vi "Resolve IP.vi"(10 "error in (no error)":errorcluster, 11 "Address In":string) -> (2 "error out":errorcluster, 3 "U32 Address":u32 format="%08x", 5 "Address Type":T1)   [LabVIEW 2020, in "Vecto.lvlib"]
uses:
  Vecto.lvlib
  Address Type.ctl
  Resolve Address Type.vi/f8bc95ce-8757-4bea-a9a5-74e77d021f7a.vi
  <vilib>/AdvancedString/1D String Array to Delimited String.vi
  <vilib>/Utility/error.llb/Error Cluster From Error Code.vi
  <vilib>/Comparison/Equal/Equal Functor/Equal Functor.lvclass
  IP Resolver/IP Resolver.lvclass
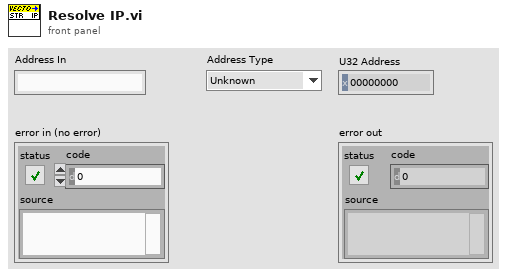
[diagram p1: front panel]
types:
  T1 = typedef "Vecto.lvlib/Address Type.ctl" = enum16{"Unknown", "Specific", "Subnet", "Any"}
  T2 = typedef "Vecto.lvlib/IP Resolver.lvclass/Address Type.ctl" = enum16{"Unknown", "Specific", "Subnet", "Any"}
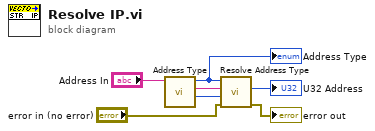
[diagram p0: block diagram]
diagram:
  n1 = call "Address Type.vi"("Address In"="Address In") -> ("Subnet Bits"=w4:i32, "Address"=w5:string, "Address Type"=w6:T2)  [unwired: 8 in]
  "Address Type" <- w6
  n2 = call "Resolve Address Type.vi"("error in (no error)"="error in (no error)", "Subnet Bits"=w4, "Address"=w5, "Address Type"=w6) -> ("error out"=→"error out":errorcluster, "U32 Address"=→"U32 Address":u32)  [unwired: 6 in]
